vi "runCtrChgAfterTime.vi"(0 "timeDif(ticks)":u32, 2 "init(ticks)":u32, 4 "forceReset":bool) -> (14 "change":bool)   [LabVIEW 2014]
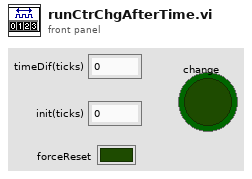
[diagram p1: front panel]
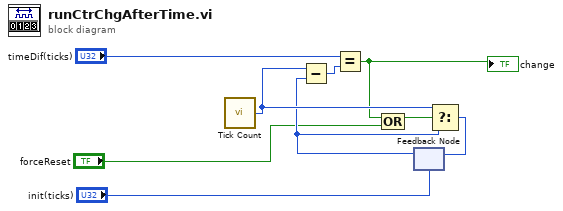
[diagram p0: block diagram]
diagram:
  n1 = call "Tick Count"() -> ("Tick Count(Ticks)"=w9:u32)
  n2 = feedback #1("init(ticks)") -> (w3:u32)
  n3 = Subtract(x=w9, y=w3) -> (x-y=w7:u32)
  n4 = Equal?(x="timeDif(ticks)", y=w7) -> (x = y?=w6:bool)
  "change" <- w6
  n5 = Compound Arithmetic op=OR(w6, "forceReset") -> (w2:bool)
  n6 = Select(t=w9, s=w2, f=w3) -> (s? t:f=w8:u32)
  n7 = feedback-in #1(w8) -> ()
